vi "Lab02.vi"() -> ()   [LabVIEW 2022 SP3]
panel:
  out "Array":i32[](array[numeric])
  out "Numeric":i32
  in  "Go":bool
  in  "Stop":bool
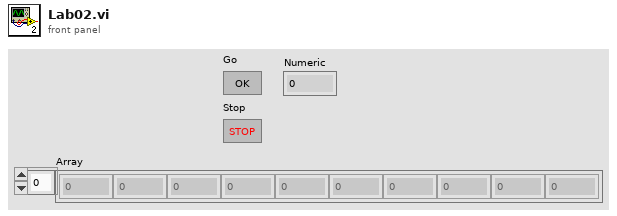
[diagram p1: front panel]
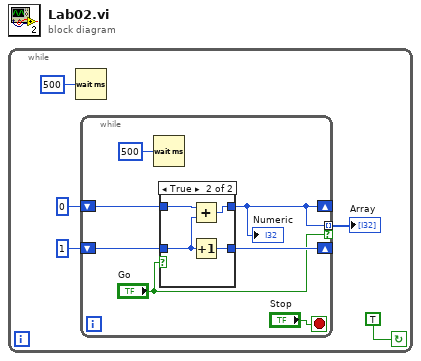
[diagram p0: block diagram]
diagram:
  n1 = while {
    stop <- TRUE continue-if-true
    n2 = Wait (ms)(milliseconds to wait=u32 500) -> ()  [unwired: 1 out]
    n3 = while {
      shift-right: [w7] -> _
      shift-left: 0 -> [w8]
      shift-right: [w9] -> _
      shift-left: 1 -> [w10]
      tunnel: [w7] -> w1 mode=indexing if="Go"
      stop <- "Stop" stop-if-true
      n4 = Wait (ms)(milliseconds to wait=u32 500) -> ()  [unwired: 1 out]
      n5 = case shown="True" "Go" {
        tunnel: w8 -> [w14 w18]
        tunnel: [w14 w15] -> w7
        tunnel: w10 -> [w13 w17]
        tunnel: [w13 w16] -> w9
        frame False {
        }
        frame True {
          n6 = Add(x=w18, y=w17) -> (x+y=w15:i32)
          n7 = Increment(x=w17) -> (x+1=w16:i32)
        }
      }
      "Numeric" <- w7
    }
    "Array" <- w1
  }
